vi "GetSlitwidth.vi"(8 "error in (no error)":errorcluster, 10 "Slit":T1(ring), 11 "HRS_Spectrometer in":refnum<class "HRS_Spectrometer.lvclass">) -> (0 "error out":errorcluster, 3 "HRS_Spectrometer out":refnum<class "HRS_Spectrometer.lvclass">)   [LabVIEW 2023, in "HRS_Spectrometer.lvlib" / "HRS_Spectrometer.lvclass"]
uses:
  HRS_Spectrometer.lvclass
  HRS_Spectrometer.lvclass/HRS_Spectrometer.ctl
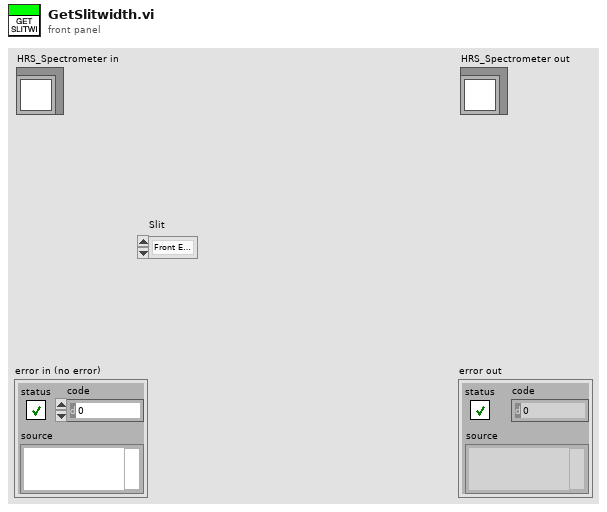
[diagram p1: front panel]
types:
  T1 = enum16{"Front Entrance Slit", "Side Entrance Slit", "Front Exit Slit", "Side Exit Slit"}
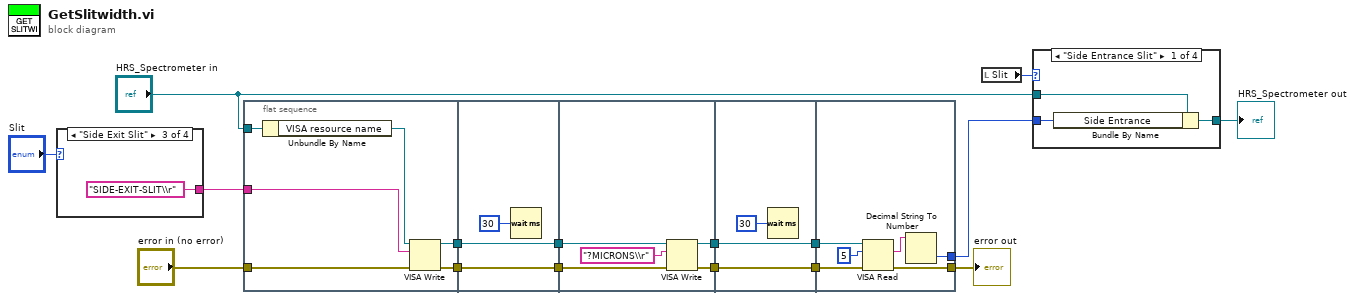
[diagram p0: block diagram]
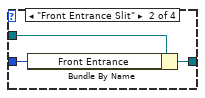
[diagram p2: hidden frame]
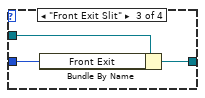
[diagram p3: hidden frame]
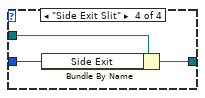
[diagram p4: hidden frame]
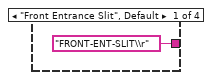
[diagram p5: hidden frame]
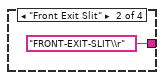
[diagram p6: hidden frame]
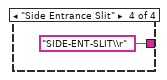
[diagram p7: hidden frame]
diagram:
  n1 = case shown="\"Side Exit Slit\"" "Slit" {
    tunnel: ["FRONT-ENT-SLIT\\r" "FRONT-EXIT-SLIT\\r" "SIDE-EXIT-SLIT\\r" "SIDE-ENT-SLIT\\r"] -> w15
    frame "Front Entrance Slit", Default {
    }
    frame "Front Exit Slit" {
    }
    frame "Side Exit Slit" {
    }
    frame "Side Entrance Slit" {
    }
  }
  n2 = flat-sequence {
    tunnel: "HRS_Spectrometer in" -> [w26]
    tunnel: w15 -> [w24]
    tunnel: [w23] -> w14
    tunnel: [w22] -> w13
    tunnel: "error in (no error)" -> [w21]
    tunnel: w14 -> [w29]
    tunnel: w13 -> [w28]
    tunnel: [w29] -> w12
    tunnel: [w28] -> w11
    tunnel: w12 -> [w33]
    tunnel: w11 -> [w34]
    tunnel: [w31] -> w5
    tunnel: [w30] -> w1
    tunnel: w5 -> [w36]
    tunnel: [w36] -> w4
    tunnel: [w35] -> w2
    tunnel: w1 -> [w35]
    tunnel: [w41] -> w6
    tunnel: [w40] -> w3
    tunnel: w4 -> [w39]
    tunnel: w2 -> [w38]
    frame #0 {
      n3 = Unbundle By Name(w26) -> ("VISA resource name"=w25:refnum<visa-resource-name>)
      n4 = VISA Write(VISA resource name=w25, write buffer=w24, error in (no error)=w21) -> (VISA resource name out=w23:refnum<visa-resource-name>, error out=w22:errorcluster)  [unwired: 1 out]
    }
    frame #1 {
      n5 = Wait (ms)(milliseconds to wait=u32 30) -> ()  [unwired: 1 out]
    }
    frame #2 {
      n6 = VISA Write(VISA resource name=w33, write buffer="?MICRONS\\r", error in (no error)=w34) -> (VISA resource name out=w30:refnum<visa-resource-name>, error out=w31:errorcluster)  [unwired: 1 out]
    }
    frame #3 {
      n7 = Wait (ms)(milliseconds to wait=u32 30) -> ()  [unwired: 1 out]
    }
    frame #4 {
      n8 = VISA Read(VISA resource name=w38, byte count=u32 5, error in (no error)=w39) -> (read buffer=w43:string, error out=w40:errorcluster)  [unwired: 2 out]
      n9 = Decimal String To Number(string=w43) -> (number=w41:i32)  [unwired: 2 in, 1 out]
    }
  }
  n10 = local read "Slit"() -> (w9:T1)
  n11 = case shown="\"Side Entrance Slit\"" w9 {
    tunnel: "HRS_Spectrometer in" -> [w46 w49 w52 w55]
    tunnel: w6 -> [w45 w48 w51 w54]
    tunnel: [w44 w47 w50 w53] -> w8
    frame "Side Entrance Slit" {
      n12 = Bundle By Name(cluster=w46, "Side Entrance"=w45) -> (w44:refnum<class "HRS_Spectrometer.lvclass">)
    }
    frame "Front Entrance Slit" {
      n13 = Bundle By Name(cluster=w49, "Front Entrance"=w48) -> (w47:refnum<class "HRS_Spectrometer.lvclass">)
    }
    frame "Front Exit Slit" {
      n14 = Bundle By Name(cluster=w52, "Front Exit"=w51) -> (w50:refnum<class "HRS_Spectrometer.lvclass">)
    }
    frame "Side Exit Slit" {
      n15 = Bundle By Name(cluster=w55, "Side Exit"=w54) -> (w53:refnum<class "HRS_Spectrometer.lvclass">)
    }
  }
  "HRS_Spectrometer out" <- w8
  "error out" <- w3
